vi "Get regeneration.vi"(8 "error in (no error)":errorcluster, 11 "NI Digital Output in":refnum<class "NI Digital Output.lvclass">) -> (0 "error out":errorcluster, 2 "regeneration":bool, 3 "NI Digital Output out":refnum<class "NI Digital Output.lvclass">)   [LabVIEW 2020, in "NI DAQmx.lvlib" / "NI Digital Output.lvclass"]
uses:
  NI Digital Output.lvclass
  NI Digital Output.lvclass/NI Digital Output.ctl
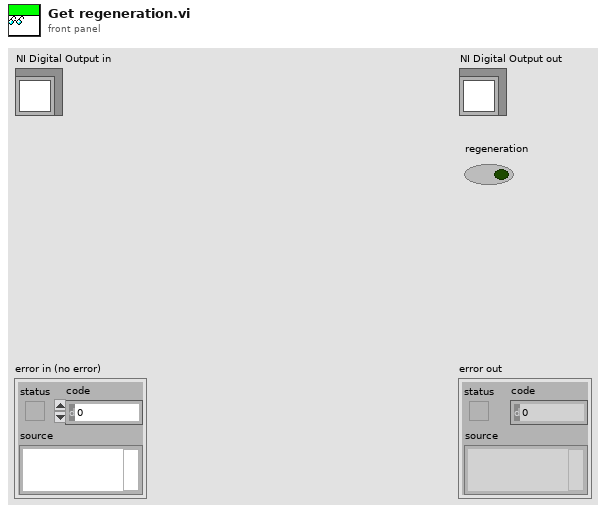
[diagram p1: front panel]
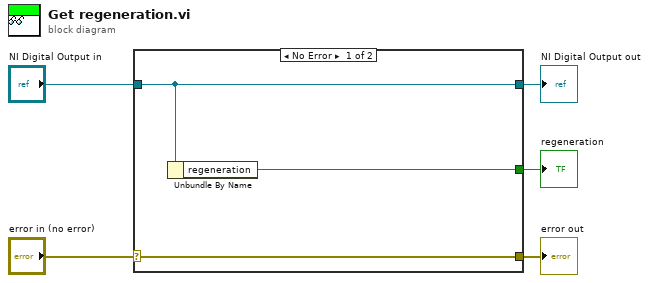
[diagram p0: block diagram]
diagram:
  n1 = case shown="No Error" "error in (no error)" {
    selector: "error in (no error)" -> [w8 w9]
    tunnel: [w8 w9] -> w4
    tunnel: [w7 w10] -> w2
    tunnel: "NI Digital Output in" -> [w7 w10]
    tunnel: [w6 _] -> w1
    frame No Error {
      n2 = Unbundle By Name(w7) -> ("regeneration"=w6:bool)
    }
    frame Error {
    }
  }
  "error out" <- w4
  "NI Digital Output out" <- w2
  "regeneration" <- w1
